vi "Dlg-Edit-Operation.vi"(8 "error in (no error)":errorcluster, 9 "Parameters":T1, 10 "Key":i32, 11 "Operations in":refnum<class "Operations.lvclass">) -> (0 "error out":errorcluster, 2 "Canceled":bool, 3 "Operations out":refnum<class "Operations.lvclass">)   [LabVIEW 2012]
uses:
  Operation/Operation Type Enum.ctl
  controls/Currencies.ctl
  Operations.lvclass
  Operation/Operation Parameters.ctl
panel:
  in  "Currency":T3
  in  "Montant":dbl
  in  "Type d'opération":T2
  in  "Add":bool
  in  "Date":timestamp format="%<%X\n%x>T"
  in  "Commentaires":string
  in  "Cancel Button":bool
  in  "Help":bool
  # "Nouveau Portefeuille"
  # "Editer une Opération"
  # "Opération"
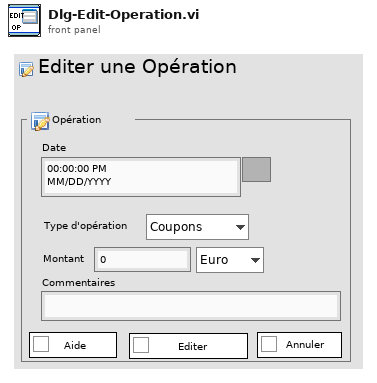
[diagram p1: front panel]
types:
  T1 = typedef "Operation Parameters.ctl" = cluster{"Date":timestamp, "Operation Type":T2, "Amount":dbl, "Comment":string, "Currency":T3}
  T2 = typedef "Operation Type Enum.ctl" = enum16{"Coupons", "Dépot", "Retrait", "Intérêts", "Taxe"}
  T3 = typedef "Currencies.ctl" = enum16{"Euro", "Dollar", "Yen", "RIM", "CHF"}
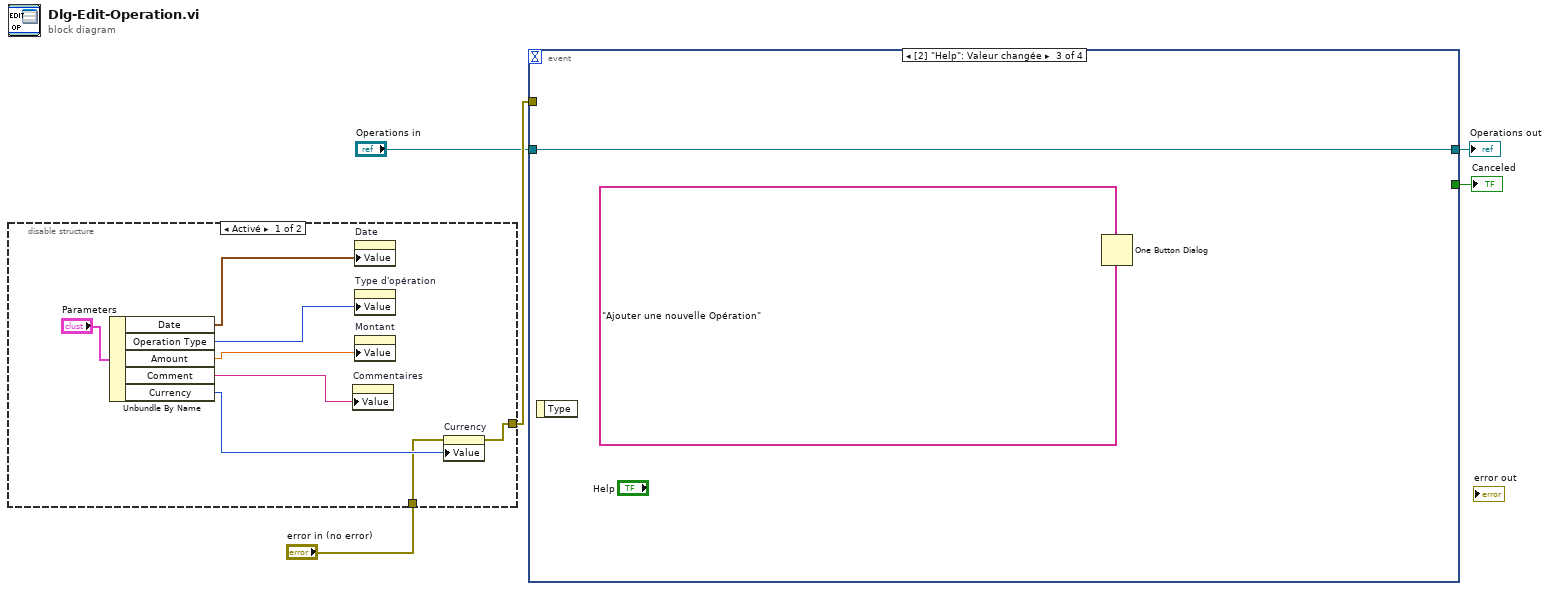
[diagram p0: block diagram]
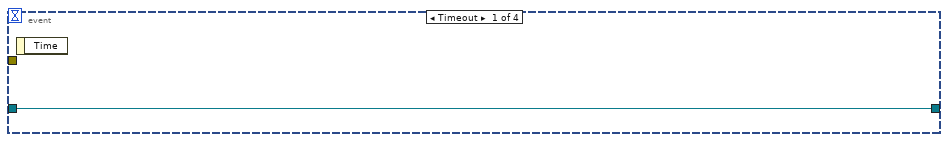
[diagram p3: hidden frame]
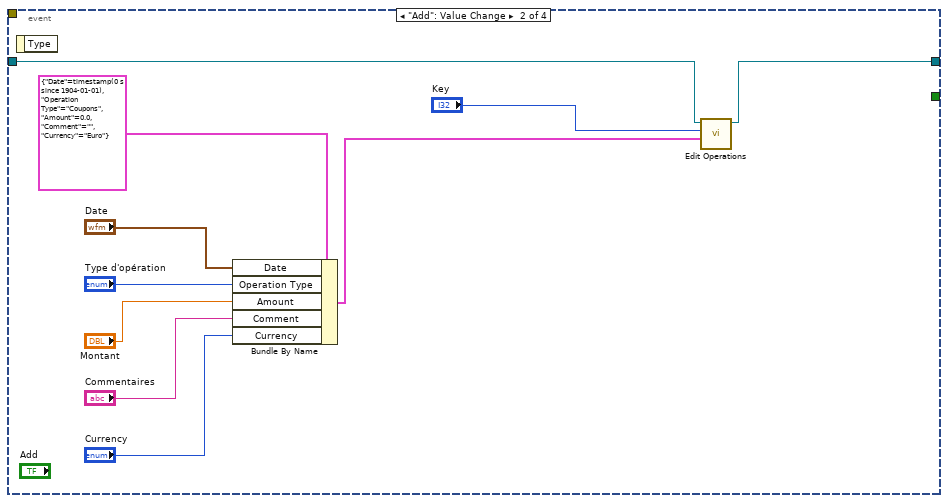
[diagram p4: hidden frame]
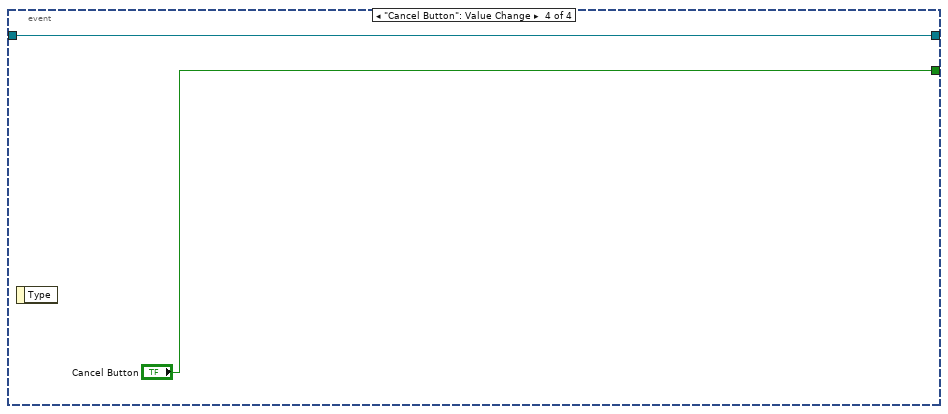
[diagram p5: hidden frame]
diagram:
  n1 = disable-structure shown="Activé" {
    disable-tunnel: [w6 _] -> w5
    disable-tunnel: "error in (no error)" -> [w7 _]
    frame Enabled {
      n2 = Unbundle By Name("Parameters") -> ("Date"=w12:timestamp, "Operation Type"=w11:T2, "Amount"=w10:dbl, "Comment"=w9:string, "Currency"=w8:T3)
      n3 = property on="Commentaires" class="Ch"("Value"=w9) -> ()  [unwired: 2 in, 2 out]
      n4 = property on="Date" class="TempsAbs (strict)"("Value"=w12) -> ()  [unwired: 2 in, 2 out]
      n5 = property on="Type d'opération" class="Énum (strict)"("Value"=w11) -> ()  [unwired: 2 in, 2 out]
      n6 = property on="Montant" class="NumNb (strict)"("Value"=w10) -> ()  [unwired: 2 in, 2 out]
      n7 = property on="Currency" class="Énum (strict)"(error in=w7, "Value"=w8) -> (error out=w6:errorcluster)  [unwired: 1 in, 1 out]
    }
    frame Disabled {
    }
  }
  n8 = event shown="[2] \"Help\": Valeur changée" {
    selector: _ -> [_ _ _ _]
    dyn-events: _ -> [_ _ _ _]
    timeout: _ -> [_ _ _ _]
    tunnel: w5 -> [_ _ _ _]
    tunnel: [_ _ _ "Cancel Button"] -> w3
    tunnel: "Operations in" -> [w14 w18 w25 w27]
    tunnel: [w14 w17 w25 w27] -> w1
    event Timeout {
      n9 = event-data() -> ()  [unwired: 1 in, 1 out]
    }
    event "Add": Value Change {
      n10 = event-data() -> ()  [unwired: 1 in, 1 out]
      n11 = Bundle By Name(cluster=T1 {"Date"=timestamp(0 s since 1904-01-01), "Operation Type"=enum."Coupons", "Amount"=0.0, "Comment"="", "Currency"=enum."Euro"} ("Parameters"), "Date"="Date", "Operation Type"="Type d'opération", "Amount"="Montant", "Comment"="Commentaires", "Currency"="Currency") -> (w16:T1)
      n12 = call "Edit Operations.vi"("Parameters"=w16, "Key"="Key", "Operations en entrée"=w18) -> ("Operations en sortie"=w17:refnum<class "Operations.lvclass">)  [unwired: 6 in, 2 out]
    }
    event "Help": Value Change {
      n13 = event-data() -> ()  [unwired: 1 in, 1 out]
      n14 = One Button Dialog(message="Ajouter une nouvelle Opération") -> ()  [unwired: 1 in, 1 out]
    }
    event "Cancel Button": Value Change {
      n15 = event-data() -> ()  [unwired: 1 in, 1 out]
    }
  }
  "Canceled" <- w3
  "Operations out" <- w1
